vi "Check Condition.vi"(8 "error in":errorcluster, 11 "File Splitting Logger in":refnum<class "File Splitting Logger.lvclass">) -> (0 "error out":errorcluster, 2 "Condition":bool, 3 "File Splitting Logger out":refnum<class "File Splitting Logger.lvclass">)   [LabVIEW 2020, in "File Splitting Logger.lvclass"]
uses:
  File Splitting Logger.lvclass
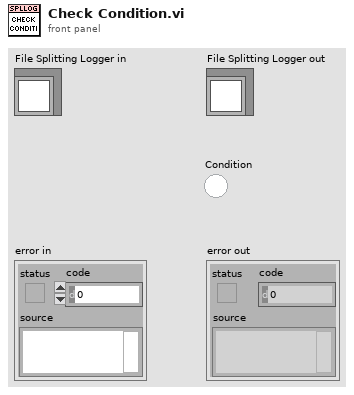
[diagram p1: front panel]
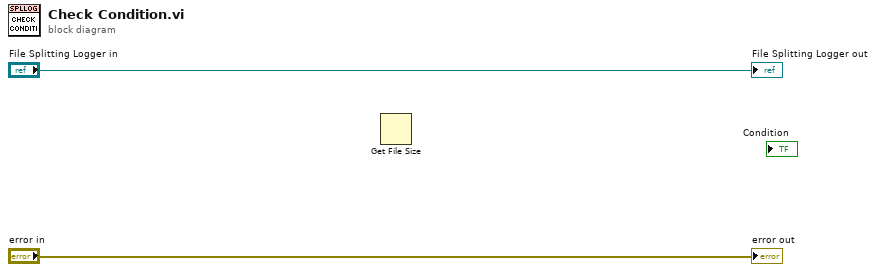
[diagram p0: block diagram]
diagram:
  n1 = Get File Size() -> ()  [unwired: 2 in, 3 out]
  "error out" <- "error in"
  "File Splitting Logger out" <- "File Splitting Logger in"
